vi "terminate.vi"(8 "error in (no error)":errorcluster, 11 "GenericPlugin in":refnum<class "GenericDAQ.lvclass">) -> (0 "error out":errorcluster, 3 "GenericPlugin out":refnum<class "GenericDAQ.lvclass">)   [LabVIEW 2010, in "GenericDAQ.lvclass"]
doc: "The dynamic dispatch version of this VI terminates the plug-in object by releasing all of its resources."
uses:
  GenericDAQ.lvclass
  GenericDAQ.lvclass/GenericDAQ.ctl
  common/classes/GenericToplevelComponent/GenericToplevelComponent/GenericToplevelComponent.lvclass
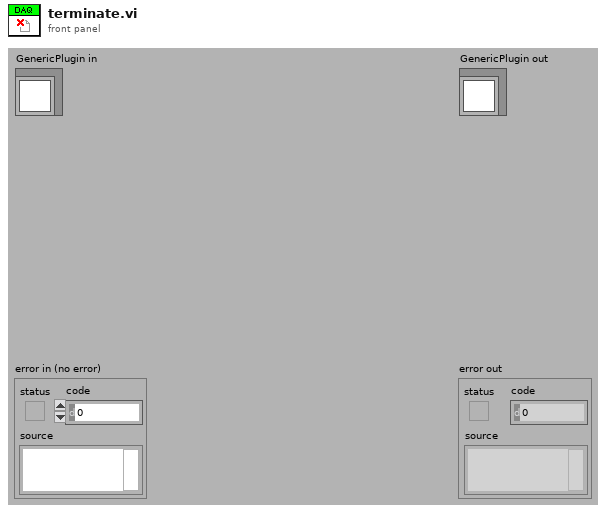
[diagram p1: front panel]
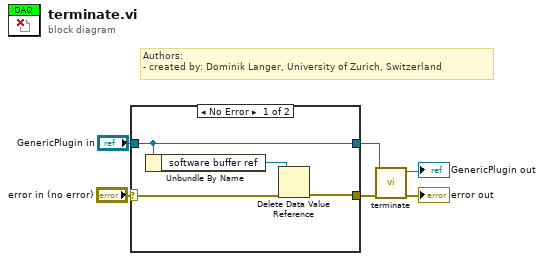
[diagram p0: block diagram]
diagram:
  # "Authors: \n- created by: Dominik Langer, University of Zurich, Switzerland"
  n1 = case shown="No Error" "error in (no error)" {
    selector: "error in (no error)" -> [w9 w12]
    tunnel: "GenericPlugin in" -> [w7 w11]
    tunnel: [w8 w12] -> w4
    tunnel: [w7 w11] -> w1
    frame No Error {
      n2 = Unbundle By Name(w7) -> ("software buffer ref"=w10:refnum<data-value>)
      n3 = Delete Data Value Reference(data value reference=w10, error in=w9) -> (error out=w8:errorcluster)  [unwired: 1 out]
    }
    frame Error {
    }
  }
  n4 = call-parent "terminate.vi"("error in (no error)"=w4, "GenericPlugin in"=w1) -> ("error out"=→"error out":errorcluster, "GenericPlugin out"=→"GenericPlugin out":refnum<class "GenericDAQ.lvclass">)  [unwired: 8 in]
